vi "Set Overload Protection.vi"(8 "error in (no error)":errorcluster, 10 "Protection ON/OFF":bool, 11 "ESM303 in":refnum<class "ESM303.lvclass">) -> (0 "error out":errorcluster, 3 "ESM303 out":refnum<class "ESM303.lvclass">)   [LabVIEW 2018, in "ESM303.lvlib" / "ESM303.lvclass"]
uses:
  ESM303.lvclass
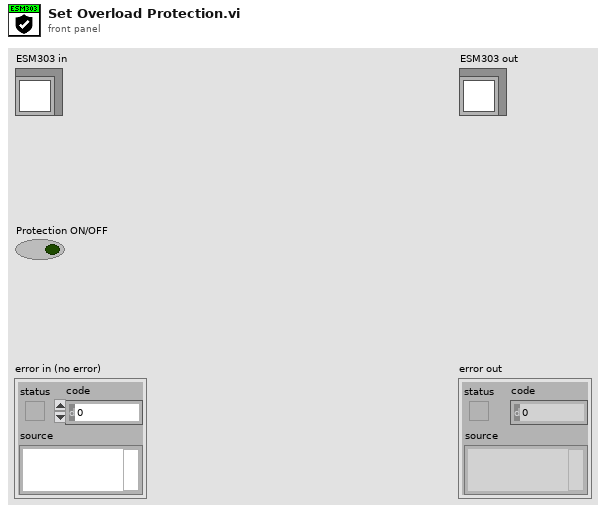
[diagram p1: front panel]
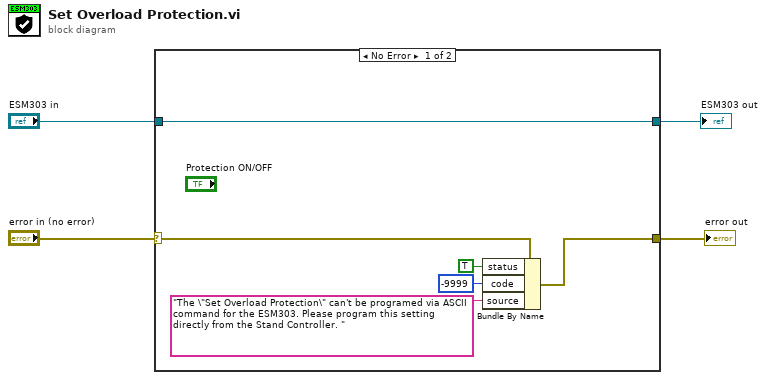
[diagram p0: block diagram]
diagram:
  n1 = case shown="No Error" "error in (no error)" {
    selector: "error in (no error)" -> [w10 w12]
    tunnel: [w9 w12] -> w3
    tunnel: [w8 w11] -> w2
    tunnel: "ESM303 in" -> [w8 w11]
    frame No Error {
      n2 = Bundle By Name(cluster=w10, "status"=TRUE, "code"=-9999, "source"="The \"Set Overload Protection\" can't be programed via ASCII command for the ESM303. Please program this setting directly from the Stand Controller. ") -> (w9:errorcluster)
    }
    frame Error {
    }
  }
  "error out" <- w3
  "ESM303 out" <- w2
